vi "VI Server_GetClusterControlRefs.vi"(7 "ClusterLabelArray":string[](array[string]), 8 "error in":errorcluster, 11 "VI Server Cluster":T1) -> (0 "error out":errorcluster, 1 "ClusterControl.Refs":refnum<vi>[](array[refnum]), 2 "ClusterControl.Labels":string[](array[string]), 3 "VI Server Cluster.OUT":T1={"Labels"=["Label", "Size", "Font", "Heght", "Width", "Ledding Denominator", "Ledding Nominator", "Label Number", "Microstep Resolution", "X", "Y", "Z", "Italic?", "Underlined?"], "Refs"=[], "VI Ref"=refnum})   [LabVIEW 2020, in "VI Server Toolkit LV2013.lvlib"]
doc: "Returns contents of the specified clusters:\n1. Controls Label;\n2. Controls Reference."
uses:
  VI Server Toolkit LV2013.lvlib
  VI Server_TypeDefs/VI Server_RefsCluster.ctl
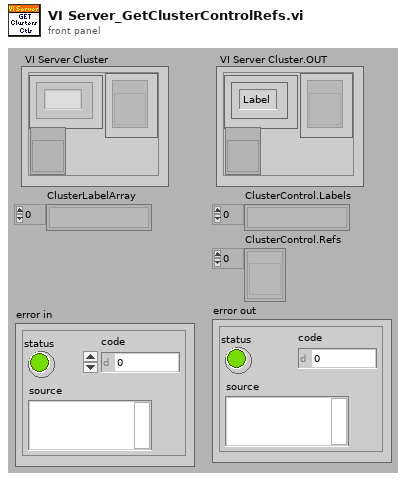
[diagram p1: front panel]
types:
  T1 = typedef "VI Server_RefsCluster.ctl" = cluster{"Labels":string[], "Refs":refnum<vi>[], "VI Ref":refnum<vi>}
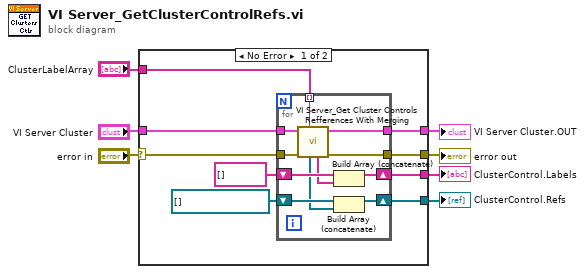
[diagram p0: block diagram]
diagram:
  n1 = case shown="No Error" "error in" {
    selector: "error in" -> [w8 w28]
    tunnel: [w16 _] -> w7
    tunnel: [w15 _] -> w6
    tunnel: "ClusterLabelArray" -> [w12 _]
    tunnel: [w11 _] -> w4
    tunnel: "VI Server Cluster" -> [w10 _]
    tunnel: [w9 w28] -> w2
    frame No Error {
      n2 = for {
        tunnel: w8 -> [w27]
        tunnel: [w26] -> w9
        tunnel: w10 -> [w25]
        tunnel: [w24] -> w11
        tunnel: w12 -> [w23] mode=indexing
        shift-right: [w21] -> w16
        shift-left: string[] [] ("ClasterControlLabels") -> [w22]
        shift-right: [w18] -> w15
        shift-left: refnum<vi>[] [] ("ClasterControRefs") -> [w19]
        n3 = call "VI Server_Get Cluster Controls Refferences With Merging.vi"("Cluster Label"=w23, "error in"=w27, "VI Server Cluster"=w25) -> ("error out"=w26:errorcluster, "VI Server Cluster.DUP"=w24:T1, "Claster.ControlLabels"=w20:string[], "Claster.ControRefs"=w17:refnum<vi>[])  [unwired: 5 out]
        n4 = Build Array (concatenate)(w22, w20) -> (w21:string[])
        n5 = Build Array (concatenate)(w19, w17) -> (w18:refnum<vi>[])
      }
    }
    frame Error {
    }
  }
  "ClusterControl.Labels" <- w7
  "ClusterControl.Refs" <- w6
  "VI Server Cluster.OUT" <- w4
  "error out" <- w2
